vi "Benchmark SV Send  LV2012 - NI Verified - 10 Byte - PC - 1Var.vi"() -> ()   [LabVIEW 2015]
panel:
  out "10 byte":u64[](array[numeric])
  in  "Reset":bool
  out "Tries":u32
  out "Average Delay (ms)":dbl
  out "Delay (ms)":u32
  in  "stop":bool
  # "Overview:  Coding that exemplifies how to benchmark the communication of Shared Variables.\nRequirements: LabVIEW 2012 or compatible\nInstructions:\n1.  Run the \"Benchmark SV Receive LV2012 - NI Verified.vi\"\n2. Run this VI\n3. Watch the amount of time it takes to communicate\n4. Stop both VIs"
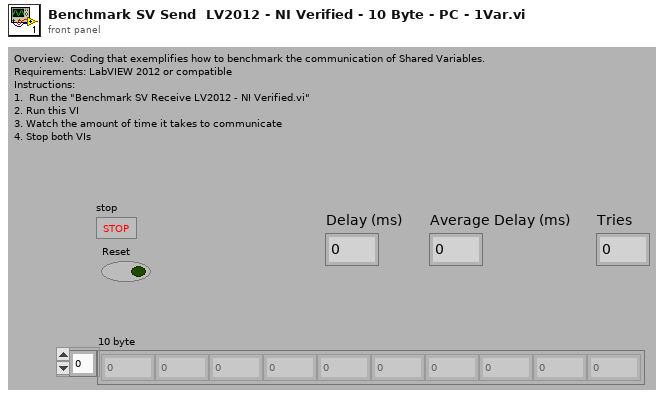
[diagram p1: front panel]
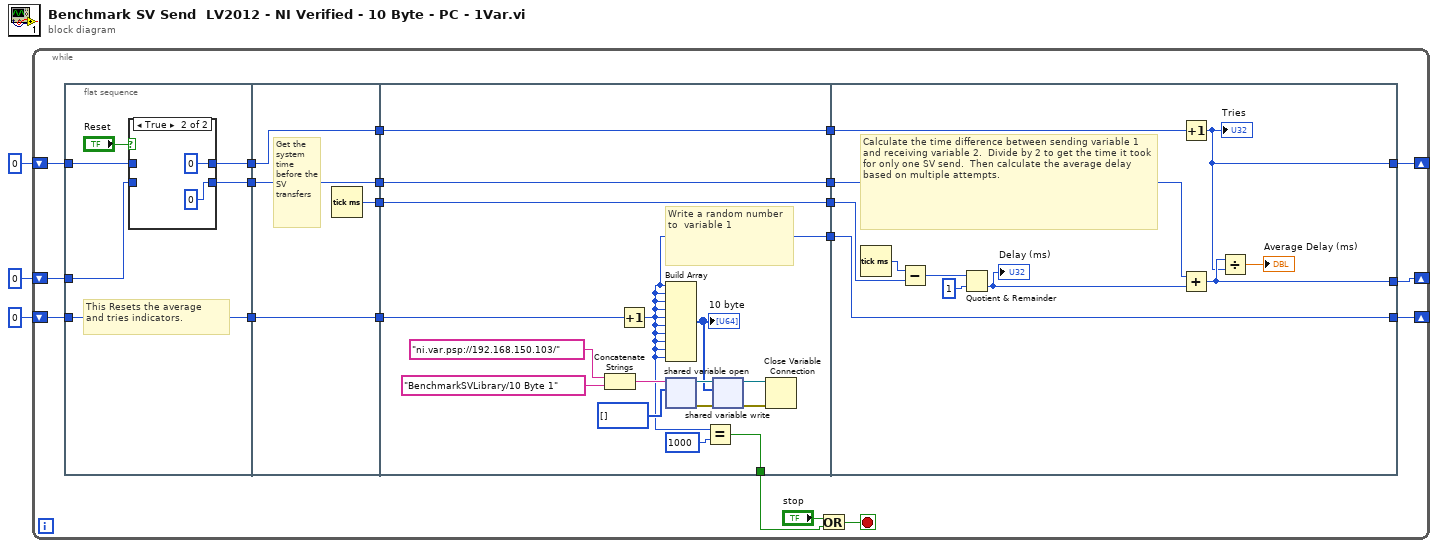
[diagram p0: block diagram]
diagram:
  n1 = while {
    shift-right: [w23] -> _
    shift-left: u32 0 -> [w15]
    shift-right: [w22] -> _
    shift-left: u32 0 -> [w16]
    shift-right: [w11] -> _
    shift-left: u64 0 -> [w12]
    stop <- w10 stop-if-true
    n2 = flat-sequence {
      tunnel: w15 -> [w29]
      tunnel: [w28] -> w20
      tunnel: [w26] -> w18
      tunnel: w16 -> [w25]
      tunnel: [w24] -> w13
      tunnel: w12 -> [w24]
      tunnel: [w35] -> w21
      tunnel: w20 -> [w37]
      tunnel: [w37] -> w19
      tunnel: w18 -> [w36]
      tunnel: [w36] -> w17
      tunnel: [w34] -> w14
      tunnel: w13 -> [w34]
      tunnel: [w53] -> w7
      tunnel: [w52] -> w6
      tunnel: [w51] -> w5
      tunnel: w21 -> [w53]
      tunnel: w19 -> [w52]
      tunnel: w17 -> [w51]
      tunnel: w14 -> [w43]
      tunnel: [w41] -> w4
      tunnel: [w39] -> w8
      tunnel: w7 -> [w63]
      tunnel: [w56] -> w23
      tunnel: w6 -> [w58]
      tunnel: [w55] -> w22
      tunnel: w5 -> [w62]
      tunnel: w4 -> [w54]
      tunnel: [w54] -> w11
      frame #0 {
        # "This Resets the average \nand tries indicators."
        n3 = case shown="True" "Reset" {
          tunnel: [w31 u32 0] -> w28
          tunnel: w29 -> [w31 _]
          tunnel: [w30 u32 0] -> w26
          tunnel: w25 -> [w30 _]
          frame False {
          }
          frame True {
          }
        }
      }
      frame #1 {
        # "Get the system time before the SV transfers"
        n4 = Tick Count (ms)() -> (millisecond timer value=w35:u32)
      }
      frame #2 {
        # "Write a random number to  variable 1"
        n5 = Concatenate Strings("ni.var.psp://192.168.150.103/" ("string"), "BenchmarkSVLibrary/10 Byte 1") -> (w46:string)
        n6 = Increment(x=w43) -> (x+1=w41:u64)
        n7 = Build Array(w41, w41, w41, w41, w41, w41, w41, w41, w41, w41) -> (w38:u64[])
        "10 byte" <- w38
        n8 = shared-variable-open(w46, u64[] [] ("appended array")) -> (w50:refnum<k21>, w47:errorcluster)  [unwired: 2 in]
        n9 = Equal?(x=w41, y=u64 1000) -> (x = y?=w39:bool)
        n10 = shared-variable-write(w50, w47, w38) -> (w48:refnum<k21>, w49:errorcluster)
        n11 = Close Variable Connection(8:w49, 11:w48) -> ()  [unwired: 1 out]
      }
      frame #3 {
        # "Calculate the time difference between sending variable 1 and receiving variable 2.  Divide by 2 to get the time it took for only one SV send.  Then calculate the average delay based on multiple attempts."
        n12 = Tick Count (ms)() -> (millisecond timer value=w64:u32)
        n13 = Subtract(x=w64, y=w63) -> (x-y=w61:u32)
        n14 = Quotient & Remainder(x=w61, y=u32 1) -> (floor(x/y)=w59:u32)  [unwired: 1 out]
        "Delay (ms)" <- w59
        n15 = Increment(x=w62) -> (x+1=w55:u32)
        "Tries" <- w55
        n16 = Add(x=w58, y=w59) -> (x+y=w56:u32)
        n17 = Divide(x=w56, y=w55) -> (x/y=→"Average Delay (ms)":dbl)
      }
    }
    n18 = Or(x="stop", y=w8) -> (x .or. y?=w10:bool)
  }
